vi "Set Timer DVR.vi"(8 "error in (no error)":errorcluster, 10 "Timer DVR":refnum<data-value>, 11 "Timed Door in":refnum<class "Timed Door.lvclass">) -> (0 "error out":errorcluster, 3 "Timed Door out":refnum<class "Timed Door.lvclass">)   [LabVIEW 2018, in "Timed Door.lvclass"]
uses:
  Timed Door.lvclass
  Timer/Timer.lvclass
  Timed Door.lvclass/Timed Door.ctl
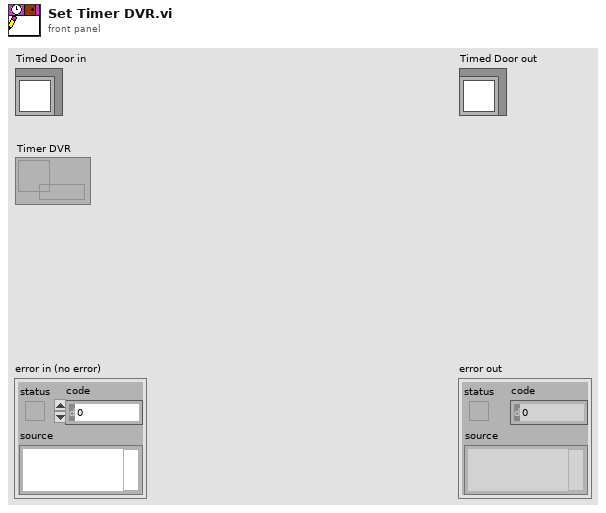
[diagram p1: front panel]
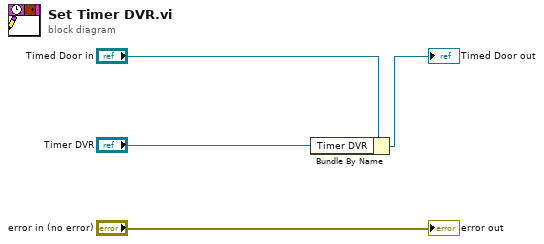
[diagram p0: block diagram]
diagram:
  n1 = Bundle By Name(cluster="Timed Door in", "Timer DVR"="Timer DVR") -> (→"Timed Door out":refnum<class "Timed Door.lvclass">)
  "error out" <- "error in (no error)"
